vi "BezahlSimulation.vi"(8 "error in":errorcluster) -> (0 "error out":errorcluster, 2 "Betrag erreicht":bool)   [LabVIEW 2023]
doc: "Bezahlsimulation\nerstellt: DI FH Mst Werner Bischof\nDatum: 22.10.2025"
uses:
  CONTROLS/fgv-status.ctl
panel:
  out "Restgeldausgabe":dbl
  in  "Storno":bool
  out "Guthaben":dbl
  out "Preis":dbl
  in  "100Euro":bool
  in  "50Euro":bool
  in  "20Euro":bool
  in  "10Euro":bool
  in  "5Euro":bool
  in  "2Euro":bool
  in  "Bezahlen":bool
  in  "1Euro":bool
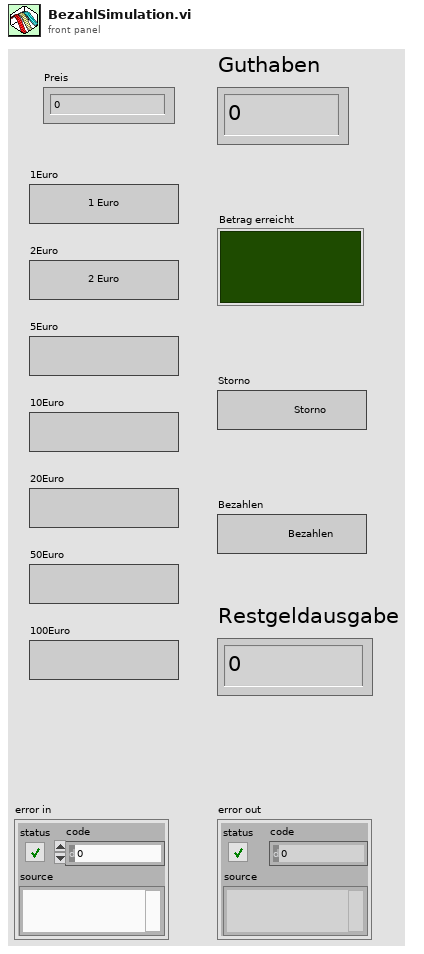
[diagram p1: front panel]
types:
  T1 = typedef "fgv-status.ctl" = enum16{"read", "write"}
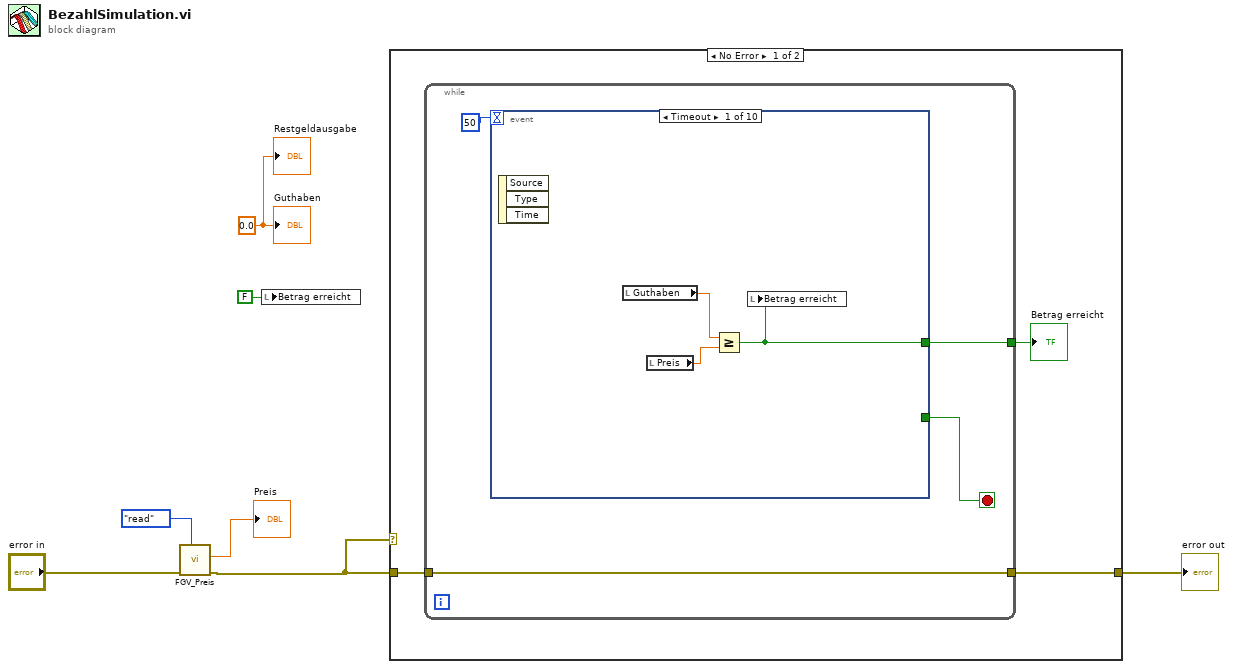
[diagram p0: block diagram]
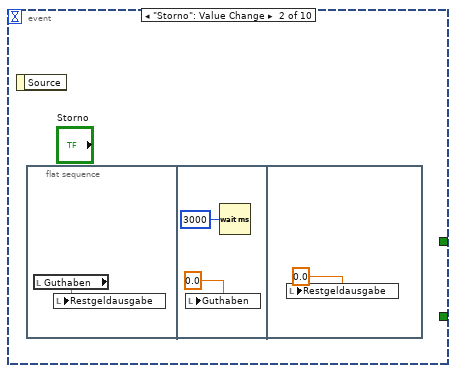
[diagram p2: hidden frame]
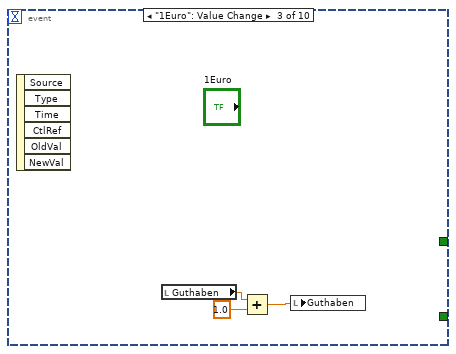
[diagram p3: hidden frame]
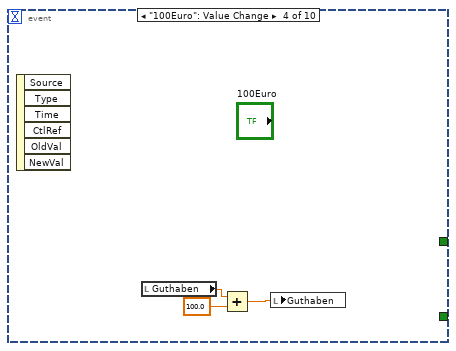
[diagram p4: hidden frame]
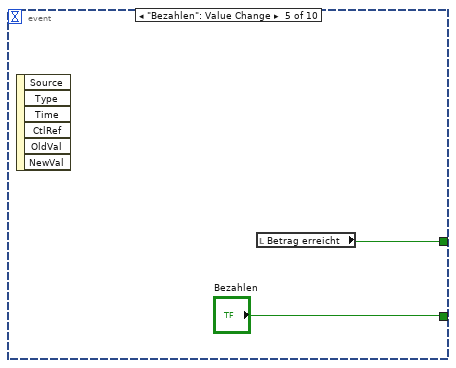
[diagram p5: hidden frame]
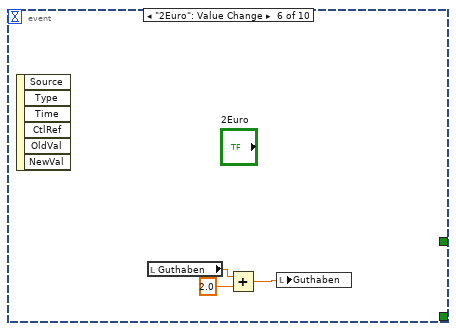
[diagram p6: hidden frame]
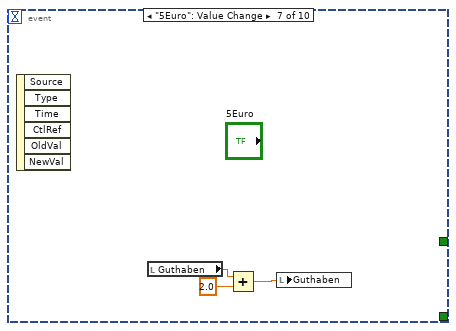
[diagram p7: hidden frame]
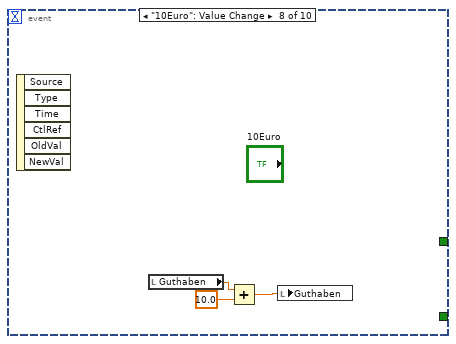
[diagram p8: hidden frame]
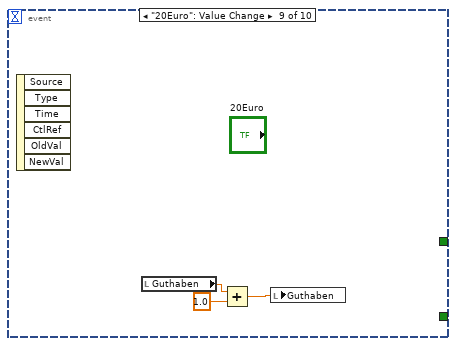
[diagram p9: hidden frame]
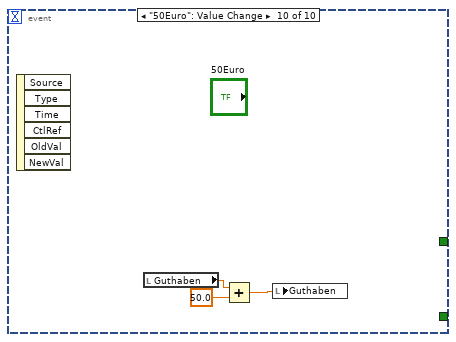
[diagram p10: hidden frame]
diagram:
  w6 = 0.0 ("Guthaben")
  n1 = call "FGV_Preis.vi"("fgv-status"=fgv-status."read", "error in"="error in") -> ("error out"=w1:errorcluster, "Preis Output"=→"Preis":dbl)  [unwired: 8 in]
  n2 = local write "Betrag erreicht"(FALSE ("Betrag erreicht")) -> ()
  n3 = case shown="No Error" w1 {
    tunnel: w1 -> [w10 w45]
    tunnel: [w9 w45] -> w5
    frame No Error {
      n4 = while {
        tunnel: [w12] -> w8
        tunnel: w10 -> [w11]
        tunnel: [w11] -> w9
        stop <- w14 stop-if-true
        n5 = event shown="[0] Timeout" {
          selector: _ -> [_ _ _ _ _ _ _ _ _ _]
          dyn-events: _ -> [_ _ _ _ _ _ _ _ _ _]
          timeout: 50 -> [_ _ _ _ _ _ _ _ _ _]
          tunnel: [_ _ _ _ "Bezahlen" _ _ _ _ _] -> w14
          tunnel: [w15 _ _ _ w28 _ _ _ _ _] -> w12
          event Timeout {
            n6 = event-data() -> ()  [unwired: 1 in, 3 out]
            n7 = local read "Guthaben"() -> (w17:dbl)
            n8 = local read "Preis"() -> (w16:dbl)
            n9 = Greater Or Equal?(x=w17, y=w16) -> (x >= y?=w15:bool)
            n10 = local write "Betrag erreicht"(w15) -> ()
          }
          event "Storno": Value Change {
            n11 = event-data() -> ()  [unwired: 1 in, 1 out]
            n12 = flat-sequence {
              frame #0 {
                n13 = local read "Guthaben"() -> (w18:dbl)
                n14 = local write "Restgeldausgabe"(w18) -> ()
              }
              frame #1 {
                n15 = local write "Guthaben"(0.0 ("Guthaben")) -> ()
                n16 = Wait (ms)(milliseconds to wait=u32 3000) -> ()  [unwired: 1 out]
              }
              frame #2 {
                n17 = local write "Restgeldausgabe"(0.0 ("Guthaben")) -> ()
              }
            }
          }
          event "1Euro": Value Change {
            n18 = event-data() -> ()  [unwired: 1 in, 6 out]
            n19 = local read "Guthaben"() -> (w24:dbl)
            n20 = Add(x=w24, y=1.0) -> (x+y=w23:dbl)
            n21 = local write "Guthaben"(w23) -> ()
          }
          event "100Euro": Value Change {
            n22 = event-data() -> ()  [unwired: 1 in, 6 out]
            n23 = local read "Guthaben"() -> (w27:dbl)
            n24 = Add(x=w27, y=100.0) -> (x+y=w26:dbl)
            n25 = local write "Guthaben"(w26) -> ()
          }
          event "Bezahlen": Value Change {
            n26 = event-data() -> ()  [unwired: 1 in, 6 out]
            n27 = local read "Betrag erreicht"() -> (w28:bool)
          }
          event "2Euro": Value Change {
            n28 = event-data() -> ()  [unwired: 1 in, 6 out]
            n29 = local read "Guthaben"() -> (w32:dbl)
            n30 = Add(x=w32, y=2.0) -> (x+y=w31:dbl)
            n31 = local write "Guthaben"(w31) -> ()
          }
          event "5Euro": Value Change {
            n32 = event-data() -> ()  [unwired: 1 in, 6 out]
            n33 = local read "Guthaben"() -> (w35:dbl)
            n34 = Add(x=w35, y=2.0) -> (x+y=w34:dbl)
            n35 = local write "Guthaben"(w34) -> ()
          }
          event "10Euro": Value Change {
            n36 = event-data() -> ()  [unwired: 1 in, 6 out]
            n37 = local read "Guthaben"() -> (w38:dbl)
            n38 = Add(x=w38, y=10.0) -> (x+y=w37:dbl)
            n39 = local write "Guthaben"(w37) -> ()
          }
          event "20Euro": Value Change {
            n40 = event-data() -> ()  [unwired: 1 in, 6 out]
            n41 = local read "Guthaben"() -> (w41:dbl)
            n42 = Add(x=w41, y=1.0) -> (x+y=w40:dbl)
            n43 = local write "Guthaben"(w40) -> ()
          }
          event "50Euro": Value Change {
            n44 = event-data() -> ()  [unwired: 1 in, 6 out]
            n45 = local read "Guthaben"() -> (w44:dbl)
            n46 = Add(x=w44, y=50.0) -> (x+y=w43:dbl)
            n47 = local write "Guthaben"(w43) -> ()
          }
        }
      }
      "Betrag erreicht" <- w8
    }
    frame Error {
    }
  }
  "error out" <- w5
  "Guthaben" <- w6
  "Restgeldausgabe" <- w6
